vi "Activate GUI Panel.vi"(8 "error in (no error)":errorcluster, 9 "banner ref":refnum<vi>, 11 "gui notifier":refnum<notifier>) -> (0 "error out":errorcluster)   [LabVIEW 2020]
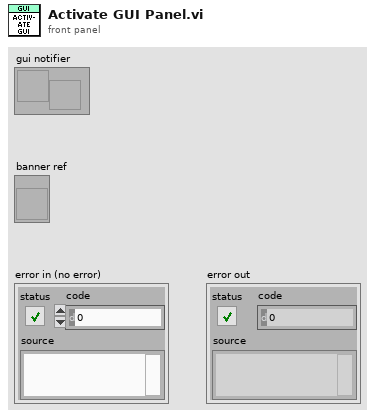
[diagram p1: front panel]
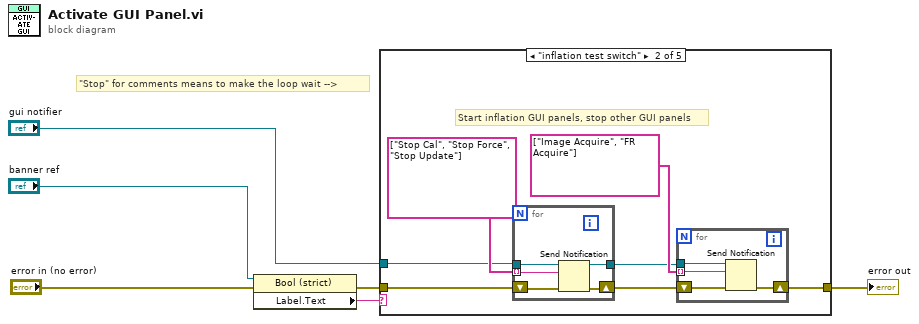
[diagram p0: block diagram]
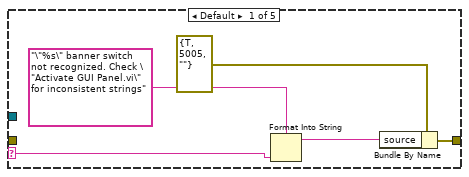
[diagram p2: hidden frame]
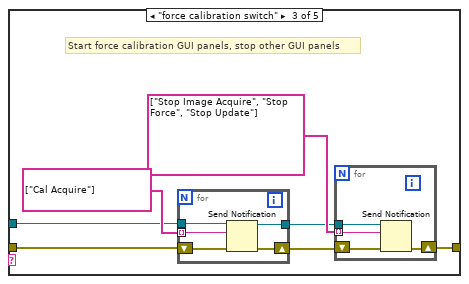
[diagram p3: hidden frame]
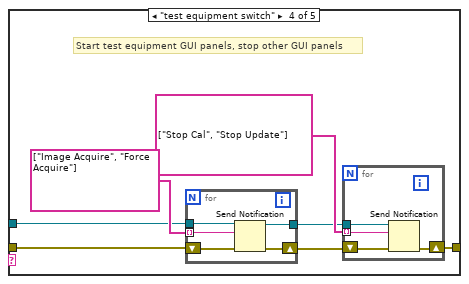
[diagram p4: hidden frame]
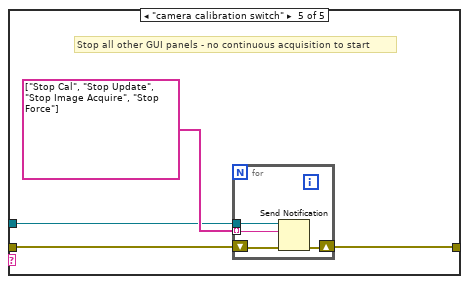
[diagram p5: hidden frame]
diagram:
  # "\"Stop\" for comments means to make the loop wait -->"
  n1 = property class="Bool (strict)"(reference="banner ref", error in="error in (no error)") -> (error out=w3:errorcluster, "Label.Text"=w6:string)  [unwired: 1 out]
  n2 = case shown="\"inflation test switch\"" w6 {
    selector: w6 -> [w7 _ _ _ _]
    tunnel: w3 -> [_ w16 w29 w46 w61]
    tunnel: [w8 w13 w28 w44 w60] -> w4
    tunnel: "gui notifier" -> [_ w15 w30 w45 w62]
    frame Default {
      n3 = Format Into String(format string="\"%s\" banner switch not recognized. Check \"Activate GUI Panel.vi\" for inconsistent strings", w7) -> (resulting string=w9:string)  [unwired: 2 in, 1 out]
      n4 = Bundle By Name(cluster=errorcluster {"status"=TRUE, "code"=5005, "source"=""} ("error constant"), "source"=w9) -> (w8:errorcluster)
    }
    frame "inflation test switch" {
      # "Start inflation GUI panels, stop other GUI panels"
      n5 = for {
        shift-right: [w22] -> w14
        shift-left: w16 -> [w23]
        tunnel: string[] ["Stop Cal", "Stop Force", "Stop Update"] ("notification") -> [w21] mode=indexing
        tunnel: w15 -> [w20]
        tunnel: [w19] -> w12
        n6 = Send Notification(notification=w21, notifier=w20, error in (no error)=w23) -> (notifier out=w19:refnum<notifier>, error out=w22:errorcluster)
      }
      n7 = for {
        tunnel: w12 -> [w26]
        tunnel: string[] ["Image Acquire", "FR Acquire"] ("notification") -> [w25] mode=indexing
        shift-right: [w24] -> w13
        shift-left: w14 -> [w27]
        n8 = Send Notification(notification=w25, notifier=w26, error in (no error)=w27) -> (error out=w24:errorcluster)  [unwired: 1 out]
      }
    }
    frame "force calibration switch" {
      # "Start force calibration GUI panels, stop other GUI panels"
      n9 = for {
        tunnel: string[] ["Cal Acquire"] ("notification") -> [w42] mode=indexing
        shift-right: [w41] -> w33
        shift-left: w29 -> [w43]
        tunnel: [w40] -> w31
        tunnel: w30 -> [w39]
        n10 = Send Notification(notification=w42, notifier=w39, error in (no error)=w43) -> (notifier out=w40:refnum<notifier>, error out=w41:errorcluster)
      }
      n11 = for {
        shift-right: [w37] -> w28
        shift-left: w33 -> [w38]
        tunnel: string[] ["Stop Image Acquire", "Stop Force", "Stop Update"] ("notification") -> [w36] mode=indexing
        tunnel: w31 -> [w35]
        n12 = Send Notification(notification=w36, notifier=w35, error in (no error)=w38) -> (error out=w37:errorcluster)  [unwired: 1 out]
      }
    }
    frame "test equipment switch" {
      # "Start test equipment GUI panels, stop other GUI panels"
      n13 = for {
        tunnel: string[] ["Image Acquire", "Force Acquire"] ("notification") -> [w58] mode=indexing
        shift-right: [w57] -> w49
        shift-left: w46 -> [w59]
        tunnel: [w56] -> w47
        tunnel: w45 -> [w55]
        n14 = Send Notification(notification=w58, notifier=w55, error in (no error)=w59) -> (notifier out=w56:refnum<notifier>, error out=w57:errorcluster)
      }
      n15 = for {
        shift-right: [w53] -> w44
        shift-left: w49 -> [w54]
        tunnel: string[] ["Stop Cal", "Stop Update"] ("notification") -> [w52] mode=indexing
        tunnel: w47 -> [w51]
        n16 = Send Notification(notification=w52, notifier=w51, error in (no error)=w54) -> (error out=w53:errorcluster)  [unwired: 1 out]
      }
    }
    frame "camera calibration switch" {
      # "Stop all other GUI panels - no continuous acquisition to start"
      n17 = for {
        shift-right: [w66] -> w60
        shift-left: w61 -> [w67]
        tunnel: string[] ["Stop Cal", "Stop Update", "Stop Image Acquire", "Stop Force"] ("notification") -> [w65] mode=indexing
        tunnel: w62 -> [w64]
        n18 = Send Notification(notification=w65, notifier=w64, error in (no error)=w67) -> (error out=w66:errorcluster)  [unwired: 1 out]
      }
    }
  }
  "error out" <- w4
